vi "operaciones matematicas.vi"() -> ()   [LabVIEW 2020]
panel:
  out "Area Rombo":dbl
  in  "d":dbl
  in  "D":dbl
  out "Área Elipse (A)":dbl
  in  "Semi Eje Menor (b)":dbl(knob) scale=0.0..500.0
  in  "Semi Eje Mayor (a)":dbl(knob) scale=0.0..500.0
  # "Ejercicios con datos numéricos"
  # "LabVIEW Clase 03 - 2022"
  # "Elipse"
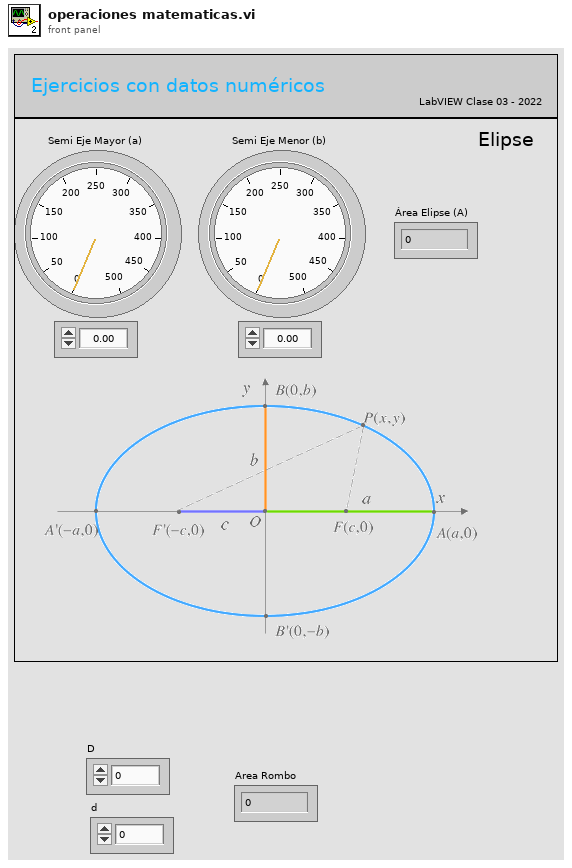
[diagram p1: front panel]
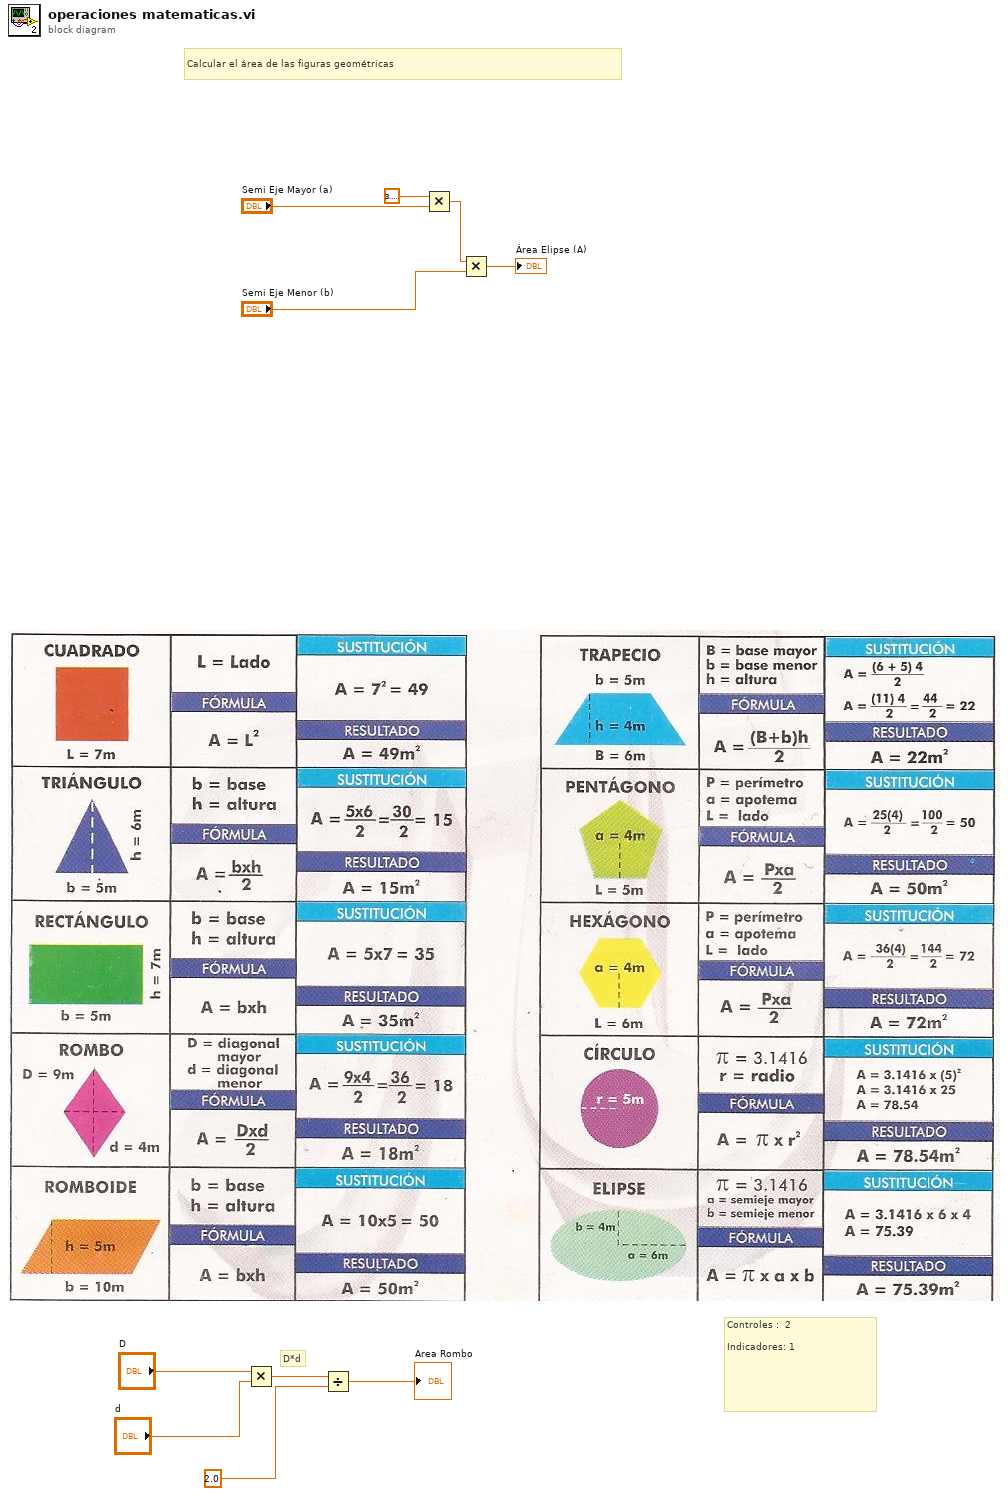
[diagram p0: block diagram]
diagram:
  # "D*d"
  # "Controles :  2\n\nIndicadores: 1"
  # "Calcular el área de las figuras geométricas"
  n1 = Multiply(x="D", y="d") -> (x*y=w3:dbl)
  n2 = Divide(x=w3, y=2.0) -> (x/y=→"Area Rombo":dbl)
  n3 = Multiply(x=3.141592653589793, y="Semi Eje Mayor (a)") -> (x*y=w8:dbl)
  n4 = Multiply(x=w8, y="Semi Eje Menor (b)") -> (x*y=→"Área Elipse (A)":dbl)
